vi "Change Message Visibility (Single).vi"(8 "error in (no error)":errorcluster, 9 "Visibility Timeout":i32, 10 "Receipt Handle":string, 11 "SQS in":refnum<class "NI_AWS_SQS.lvclass">) -> (0 "error out":errorcluster, 3 "SQS out":refnum<class "NI_AWS_SQS.lvclass">)   [LabVIEW 2015, in "NI_AWS_SQS.lvclass"]
uses:
  NI_AWS_SQS.lvclass
  Core/Name Value Pair.ctl
  Core/Request Options.ctl
  NI_AWS_SQS.lvclass/NI_AWS_SQS.ctl
  Read Account Number.vi
  Read Name.vi
  Core/NI_AWS_Core.lvclass
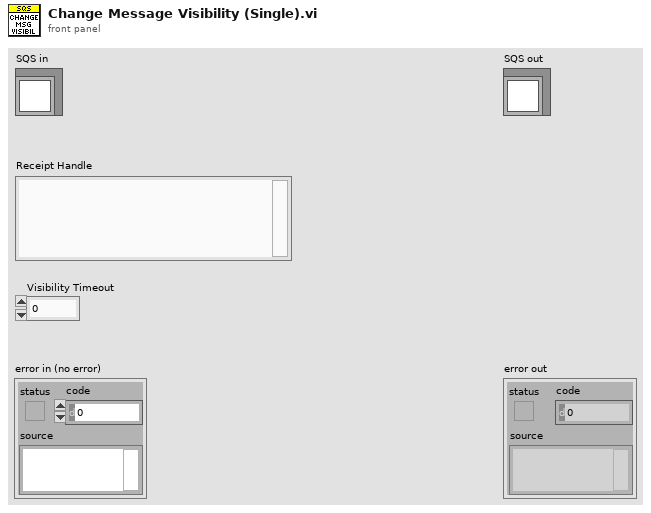
[diagram p1: front panel]
types:
  T1 = typedef "NI_AWS_Core.lvclass/Name Value Pair.ctl" = cluster{"name":string, "value":string}
  T2 = typedef "NI_AWS_Core.lvclass/Request Options.ctl" = cluster{"request headers":T1[], "request parameters":T1[], "request body":string}
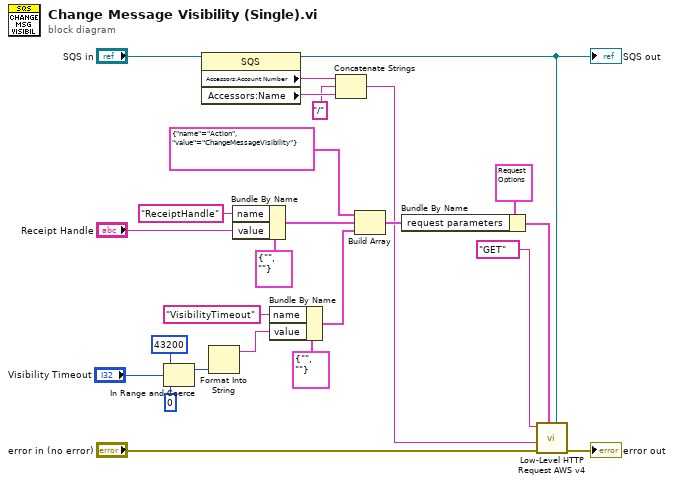
[diagram p0: block diagram]
diagram:
  n1 = In Range and Coerce(upper limit=43200, x="Visibility Timeout", lower limit=0) -> (coerced(x)=w2:i32)  [unwired: 1 out]
  n2 = property class="SQS"(reference="SQS in") -> (reference out=w18:refnum<class "NI_AWS_SQS.lvclass">, "Accessors:Account Number"=w17:string, "Accessors:Name"=w16:string)  [unwired: 1 in, 1 out]
  "SQS out" <- w18
  n3 = Format Into String(w2) -> (resulting string=w1:string)  [unwired: 3 in, 1 out]
  n4 = Bundle By Name(cluster=T1 {"name"="", "value"=""} ("element"), "name"="ReceiptHandle", "value"="Receipt Handle") -> (w11:T1)
  n5 = Bundle By Name(cluster=T1 {"name"="", "value"=""} ("element"), "name"="VisibilityTimeout", "value"=w1) -> (w6:T1)
  n6 = Concatenate Strings(w17, "/", w16) -> (w14:string)
  n7 = Build Array(T1 {"name"="Action", "value"="ChangeMessageVisibility"} ("Cluster"), w11, w6) -> (w19:T1[])
  n8 = Bundle By Name(cluster=T2 {"request headers"=[], "request parameters"=[{"name"="Action", "value"="ListQueues"}], "request body"=""} ("Request Options"), "request parameters"=w19) -> (w20:T2)
  n9 = call "Low-Level HTTP Request AWS v4.vi"("AWS Core"=w18, "Request Options"=w20, "error in (no error)"="error in (no error)", "URL Suffix"=w14, "HTTP-Verb"="GET") -> ("error out"=→"error out":errorcluster)  [unwired: 4 in, 2 out]
